vi "Set Current Calibration Gain.vi"(0 "VISA resource name":refnum<visa-resource-name>, 5 "Gain (1)":dbl=1.0, 11 "error in (no error)":errorcluster) -> (4 "VISA resource name out":refnum<visa-resource-name>, 15 "error out":errorcluster)   [LabVIEW 2020, in "NH Research Regenerative Test Series.lvlib"]
doc: "This command will cause the device to calculate and store in RAM its gain. Set Operation to battery before and during calibration. Set Regulation Gain to 0 before and during calibration. Calibrate Current Offset before calibrating Current Gain. With current at 90% of maximum, send the actual current. Values are changed in RAM only, to save permanently call Save Calibration.vi."
uses:
  NH Research Regenerative Test Series.lvlib
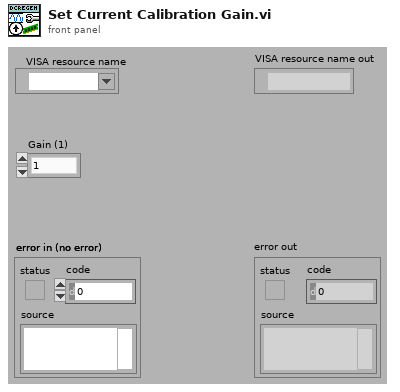
[diagram p1: front panel]
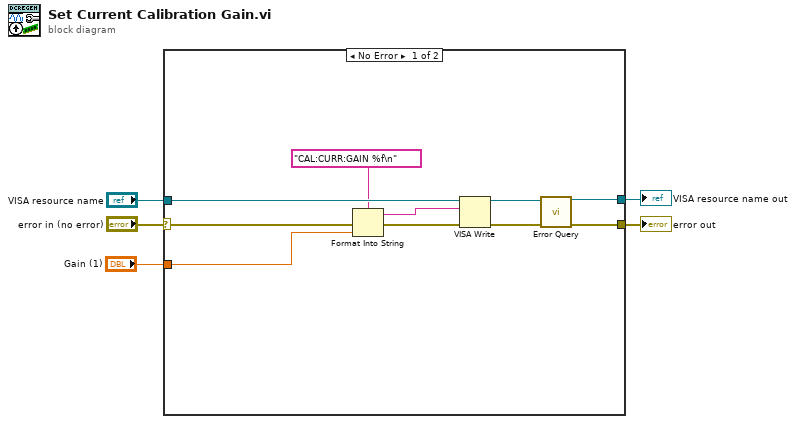
[diagram p0: block diagram]
diagram:
  n1 = case shown="No Error" "error in (no error)" {
    selector: "error in (no error)" -> [w12 w17]
    tunnel: [w13 w17] -> w4
    tunnel: [w15 w16] -> w2
    tunnel: "VISA resource name" -> [w14 w16]
    tunnel: "Gain (1)" -> [w6 _]
    frame No Error {
      n2 = Format Into String(format string="CAL:CURR:GAIN %f\n", error in=w12, w6) -> (resulting string=w9:string, error out=w11:errorcluster)  [unwired: 1 in]
      n3 = VISA Write(VISA resource name=w14, write buffer=w9, error in (no error)=w11) -> (VISA resource name out=w8:refnum<visa-resource-name>, error out=w7:errorcluster)  [unwired: 1 out]
      n4 = call "Error Query.vi"("VISA resource name"=w8, "error in (no error)"=w7) -> ("VISA resource name out"=w15:refnum<visa-resource-name>, "error out"=w13:errorcluster)  [unwired: 10 in, 2 out]
    }
    frame Error {
    }
  }
  "error out" <- w4
  "VISA resource name out" <- w2
